vi "IDS_getLockStatus.vi"(8 "error in (no error)":errorcluster, 11 "deviceHandle":i32) -> (0 "error out":errorcluster, 1 "authorized out":bool, 2 "locked out":bool, 3 "deviceHandle out":i32)   [LabVIEW 2016]
panel:
  in  "authorized":bool
  in  "locked":bool
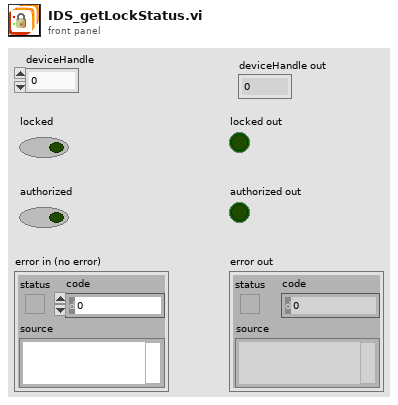
[diagram p1: front panel]
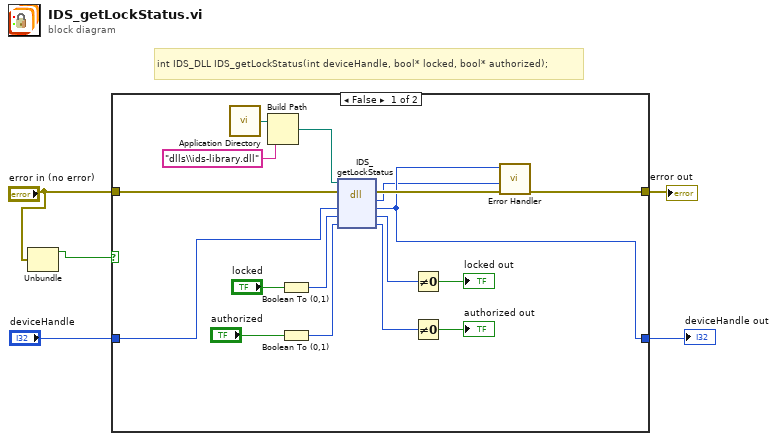
[diagram p0: block diagram]
diagram:
  # "int IDS_DLL IDS_getLockStatus(int deviceHandle, bool* locked, bool* authorized);"
  n1 = Unbundle("error in (no error)") -> ("status"=w1:bool)  [unwired: 2 out]
  n2 = case shown="False" w1 {
    tunnel: "error in (no error)" -> [w14 w24]
    tunnel: [w12 w24] -> w5
    tunnel: "deviceHandle" -> [w11 w23]
    tunnel: [w10 w23] -> w3
    frame False {
      n3 = call <vilib>:"Application Directory.vi"() -> ("Application Directory"=w8:path)
      n4 = Build Path(base path=w8, name or relative path="dlls\\ids-library.dll" ("ipAddress")) -> (appended path=w6:path)
      n5 = Boolean To (0,1)(Boolean="locked") -> (0, 1=w21:i16)
      n6 = Boolean To (0,1)(Boolean="authorized") -> (0, 1=w17:i16)
      n7 = dll-call lib="C:/Users/matheus/Desktop/LabVIEW_Draft_V1.6.0/dlls/ids-library.*" fn="IDS_getLockStatus"(path in=w6, error in=w14, "deviceHandle"=w11, "locked"=w21, "authorized"=w17) -> (error out=w13:errorcluster, "return type"=w9:i32, "deviceHandle"=w10:i32, "locked"=w19:u8, "authorized"=w15:u8)  [unwired: 1 in, 1 out]
      n8 = Not Equal To 0?(x=w19) -> (x != 0?=→"locked out":bool)
      n9 = Not Equal To 0?(x=w15) -> (x != 0?=→"authorized out":bool)
      n10 = call "Error Handler.vi"("error in (no error)"=w13, "error code"=w9, "deviceHandle"=w10) -> ("error out"=w12:errorcluster)  [unwired: 7 in, 1 out]
    }
    frame True {
    }
  }
  "error out" <- w5
  "deviceHandle out" <- w3
